vi "removeStiff.vi"() -> ()   [LabVIEW 2015]
uses:
  GlobalPath.vi
  GlobalData.vi
  GlobalVi.vi
panel:
  in  "ptfe 6":bool caption="Move the stiffback away from the panel"
  in  "ptfe 5":bool caption="Lift the stiffback from the panel"
  in  "Done ?":bool
  in  "ptfe 4":bool caption="Connect the stiffback to the movement arch"
  in  "ptfe 3":bool caption="Remove the weights placed on the panel"
  in  "ptfe 2":bool caption="Stop the table vacuum"
  # "Stiffback Removal"
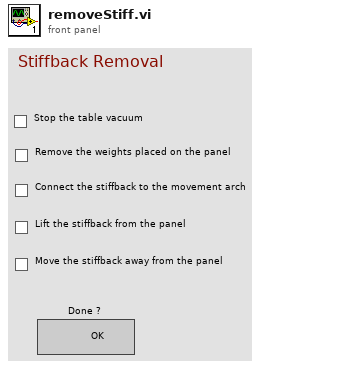
[diagram p1: front panel]
types:
  T1 = enum16{"open", "replace", "create", "open or create", "replace or create", "replace or create with confirmation"}
  T2 = enum32{"Bad", "Idle", "Run top level", "Running"}
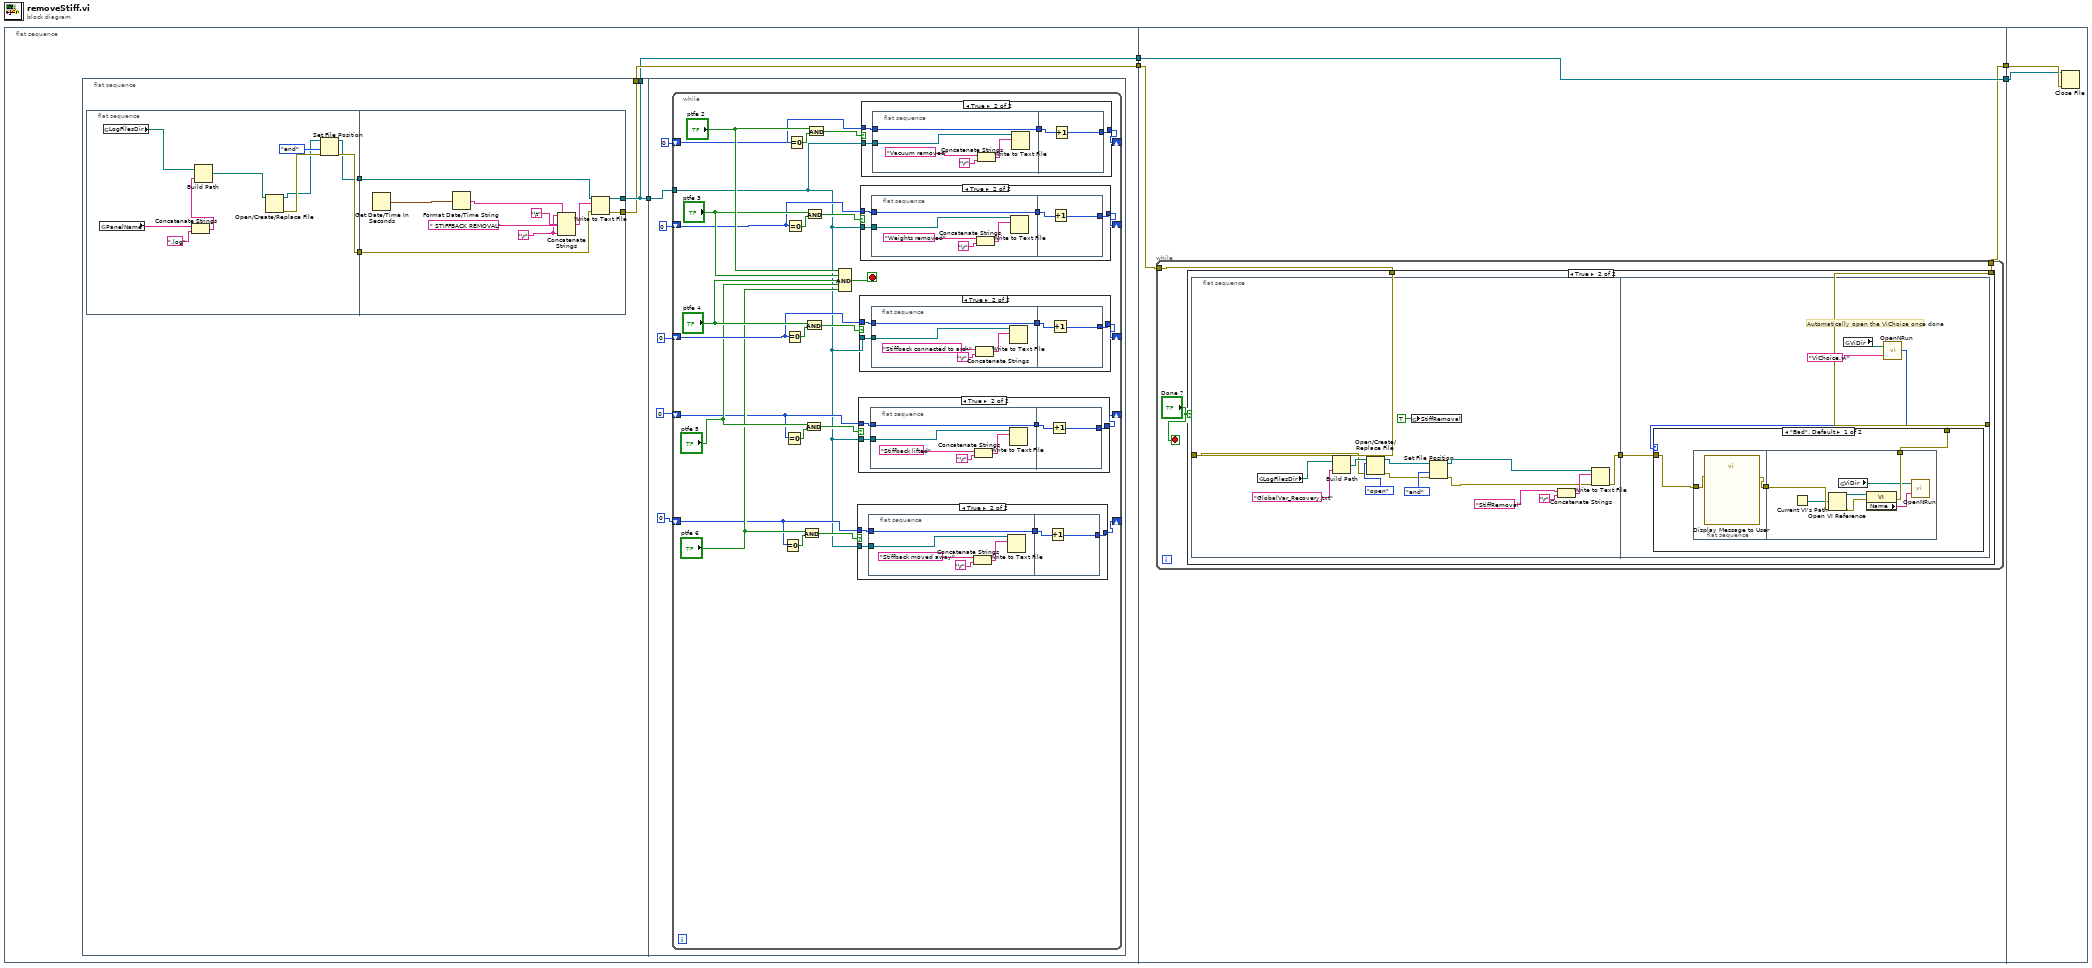
[diagram p0: block diagram]
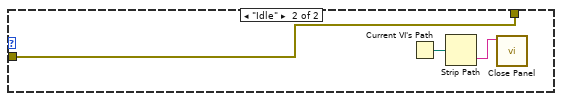
[diagram p8: hidden frame]
diagram:
  n1 = flat-sequence {
    tunnel: [w6] -> w3
    tunnel: [w5] -> w2
    tunnel: [w126] -> w4
    tunnel: w3 -> [w125]
    tunnel: w2 -> [w127]
    tunnel: [w127] -> w1
    tunnel: w4 -> [w171]
    tunnel: w1 -> [w170]
    frame #0 {
      n2 = flat-sequence {
        tunnel: [w10] -> w7
        tunnel: [w10] -> w5
        tunnel: [w9] -> w6
        tunnel: w7 -> [w37]
        frame #0 {
          n3 = flat-sequence {
            tunnel: [w13] -> w11
            tunnel: [w15] -> w8
            tunnel: w11 -> [w27]
            tunnel: [w26] -> w10
            tunnel: [w25] -> w9
            tunnel: w8 -> [w24]
            frame #0 {
              n4 = global read "GlobalData.vi" "PanelName"() -> (w20:string)
              n5 = global read "GlobalPath.vi" "LogFilesDir"() -> (w12:path)
              n6 = Concatenate Strings(w20, ".log") -> (w19:string)
              n7 = Build Path(base path=w12, name or relative path=w19) -> (appended path=w18:path)
              n8 = Open/Create/Replace File(file path (use dialog)=w18) -> (refnum out=w14:refnum<file>, error out=w16:errorcluster)  [unwired: 5 in, 1 out]
              n9 = Set File Position(refnum=w14, from (0:start)=enum16{"start", "end", "current"}."end", error in=w16) -> (refnum out=w13:refnum<file>, error out=w15:errorcluster)  [unwired: 1 in]
            }
            frame #1 {
              w22 = "\r"
              n10 = Get Date/Time In Seconds() -> (seconds since 1Jan1904=w23:timestamp)
              n11 = Format Date/Time String(seconds (now)=w23) -> (date/time string=w29:string)  [unwired: 2 in]
              n12 = Concatenate Strings(w22, w29, "\t", " STIFFBACK REMOVAL", w22) -> (w28:string)
              n13 = Write to Text File(file (use dialog)=w27, text=w28, error in=w24) -> (refnum out=w26:refnum<file>, error out=w25:errorcluster)  [unwired: 1 in, 1 out]
            }
          }
        }
        frame #1 {
          n14 = while {
            tunnel: w37 -> [w38]
            shift-right: [w55] -> _
            shift-left: 0 -> [w60]
            shift-right: [w54] -> _
            shift-left: 0 -> [w56]
            shift-right: [w49] -> _
            shift-left: 0 -> [w50]
            shift-right: [w40] -> _
            shift-left: 0 -> [w42]
            shift-right: [w39] -> _
            shift-left: 0 -> [w41]
            stop <- w64 stop-if-true
            n15 = Equal To 0?(x=w42) -> (x = 0?=w46:bool)
            n16 = Equal To 0?(x=w41) -> (x = 0?=w48:bool)
            n17 = Equal To 0?(x=w50) -> (x = 0?=w53:bool)
            n18 = Equal To 0?(x=w56) -> (x = 0?=w59:bool)
            n19 = Equal To 0?(x=w60) -> (x = 0?=w63:bool)
            n20 = And(x="ptfe 6", y=w46) -> (x .and. y?=w45:bool)
            n21 = And(x="ptfe 5", y=w48) -> (x .and. y?=w47:bool)
            n22 = And(x="ptfe 4", y=w53) -> (x .and. y?=w52:bool)
            n23 = And(x="ptfe 3", y=w59) -> (x .and. y?=w58:bool)
            n24 = And(x="ptfe 2", y=w63) -> (x .and. y?=w62:bool)
            n25 = Compound Arithmetic op=AND("ptfe 2", "ptfe 3", "ptfe 4", "ptfe 5", "ptfe 6") -> (w64:bool)
            n26 = case shown="True" w45 {
              tunnel: w38 -> [_ w69]
              tunnel: w42 -> [w65 w67]
              tunnel: [w65 w66] -> w40
              frame False {
              }
              frame True {
                n27 = flat-sequence {
                  tunnel: w69 -> [w72]
                  tunnel: [w71] -> w68
                  tunnel: w67 -> [w71]
                  tunnel: w68 -> [w76]
                  tunnel: [w75] -> w66
                  frame #0 {
                    n28 = Concatenate Strings("Stiffback moved away", "\r") -> (w74:string)
                    n29 = Write to Text File(file (use dialog)=w72, text=w74) -> ()  [unwired: 2 in, 3 out]
                  }
                  frame #1 {
                    n30 = Increment(x=w76) -> (x+1=w75:i32)
                  }
                }
              }
            }
            n31 = case shown="True" w47 {
              tunnel: w38 -> [_ w81]
              tunnel: w41 -> [w77 w79]
              tunnel: [w77 w78] -> w39
              frame False {
              }
              frame True {
                n32 = flat-sequence {
                  tunnel: w81 -> [w84]
                  tunnel: [w83] -> w80
                  tunnel: w79 -> [w83]
                  tunnel: w80 -> [w88]
                  tunnel: [w87] -> w78
                  frame #0 {
                    n33 = Concatenate Strings("Stiffback lifted", "\r") -> (w86:string)
                    n34 = Write to Text File(file (use dialog)=w84, text=w86) -> ()  [unwired: 2 in, 3 out]
                  }
                  frame #1 {
                    n35 = Increment(x=w88) -> (x+1=w87:i32)
                  }
                }
              }
            }
            n36 = case shown="True" w52 {
              tunnel: w38 -> [_ w93]
              tunnel: w50 -> [w89 w91]
              tunnel: [w89 w90] -> w49
              frame False {
              }
              frame True {
                n37 = flat-sequence {
                  tunnel: w93 -> [w96]
                  tunnel: [w95] -> w92
                  tunnel: w91 -> [w95]
                  tunnel: w92 -> [w100]
                  tunnel: [w99] -> w90
                  frame #0 {
                    n38 = Concatenate Strings("Stiffback connected to arch", "\r") -> (w98:string)
                    n39 = Write to Text File(file (use dialog)=w96, text=w98) -> ()  [unwired: 2 in, 3 out]
                  }
                  frame #1 {
                    n40 = Increment(x=w100) -> (x+1=w99:i32)
                  }
                }
              }
            }
            n41 = case shown="True" w58 {
              tunnel: w38 -> [_ w105]
              tunnel: w56 -> [w101 w103]
              tunnel: [w101 w102] -> w54
              frame False {
              }
              frame True {
                n42 = flat-sequence {
                  tunnel: w105 -> [w108]
                  tunnel: [w107] -> w104
                  tunnel: w103 -> [w107]
                  tunnel: w104 -> [w112]
                  tunnel: [w111] -> w102
                  frame #0 {
                    n43 = Concatenate Strings("Weights removed", "\r") -> (w110:string)
                    n44 = Write to Text File(file (use dialog)=w108, text=w110) -> ()  [unwired: 2 in, 3 out]
                  }
                  frame #1 {
                    n45 = Increment(x=w112) -> (x+1=w111:i32)
                  }
                }
              }
            }
            n46 = case shown="True" w62 {
              tunnel: w38 -> [_ w117]
              tunnel: w60 -> [w113 w115]
              tunnel: [w113 w114] -> w55
              frame False {
              }
              frame True {
                n47 = flat-sequence {
                  tunnel: w117 -> [w120]
                  tunnel: [w119] -> w116
                  tunnel: w115 -> [w119]
                  tunnel: w116 -> [w124]
                  tunnel: [w123] -> w114
                  frame #0 {
                    n48 = Concatenate Strings("Vacuum removed", "\r") -> (w122:string)
                    n49 = Write to Text File(file (use dialog)=w120, text=w122) -> ()  [unwired: 2 in, 3 out]
                  }
                  frame #1 {
                    n50 = Increment(x=w124) -> (x+1=w123:i32)
                  }
                }
              }
            }
          }
        }
      }
    }
    frame #1 {
      n51 = while {
        tunnel: [w129] -> w126
        tunnel: w125 -> [w128]
        stop <- "Done ?" stop-if-true
        n52 = case shown="True" "Done ?" {
          tunnel: [w131 w133] -> w129
          tunnel: w128 -> [w131 w132]
          frame False {
          }
          frame True {
            n53 = flat-sequence {
              tunnel: w132 -> [w138]
              tunnel: [w137] -> w134
              tunnel: [w151] -> w133
              tunnel: w134 -> [w150]
              frame #0 {
                n54 = global read "GlobalPath.vi" "LogFilesDir"() -> (w135:path)
                n55 = Build Path(base path=w135, name or relative path="GlobalVar_Recovery.txt") -> (appended path=w147:path)
                n56 = Open/Create/Replace File(file path (use dialog)=w147, error in=w138, operation (0:open)=T1."open") -> (refnum out=w143:refnum<file>, error out=w144:errorcluster)  [unwired: 3 in, 1 out]
                n57 = global write "GlobalVi.vi" "StiffRemoval"(TRUE) -> ()
                n58 = Set File Position(refnum=w143, from (0:start)=enum16{"start", "end", "current"}."end", error in=w144) -> (refnum out=w140:refnum<file>, error out=w139:errorcluster)  [unwired: 1 in]
                n59 = Concatenate Strings("StiffRemoval", "\r") -> (w142:string)
                n60 = Write to Text File(file (use dialog)=w140, text=w142, error in=w139) -> (error out=w137:errorcluster)  [unwired: 1 in, 2 out]
              }
              frame #1 {
                # "Automatically open the ViChoise once done"
                n61 = global read "GlobalPath.vi" "ViDir"() -> (w154:path)
                n62 = call "OpenNRun.vi"("VI name"="ViChoice.vi", "ViDirPath"=w154) -> ("Execution:State"=w153:T2)
                n63 = case shown="\"Bad\", Default" w153 {
                  tunnel: [w155 w167] -> w151
                  tunnel: w150 -> [w156 w167]
                  frame "Bad", Default {
                    n64 = flat-sequence {
                      tunnel: w156 -> [w159]
                      tunnel: [w158] -> w157
                      tunnel: [w163] -> w155
                      tunnel: w157 -> [w162]
                      frame #0 {
                        n65 = call "Display Message to User"("error in (no error)"=w159) -> ("error out"=w158:errorcluster)  [unwired: 9 in, 1 out]
                      }
                      frame #1 {
                        n66 = Current VI's Path() -> (path=w160:path)
                        n67 = Open VI Reference(vi path=w160, error in (no error)=w162) -> (vi reference=w166:refnum<vi>, error out=w165:errorcluster)  [unwired: 4 in]
                        n68 = global read "GlobalPath.vi" "ViDir"() -> (w161:path)
                        n69 = property class="VI"(reference=w166, error in=w165) -> (error out=w163:errorcluster, "Name"=w164:string)  [unwired: 1 out]
                        n70 = call "OpenNRun.vi"("VI name"=w164, "ViDirPath"=w161) -> ()  [unwired: 1 out]
                      }
                    }
                  }
                  frame "Idle" {
                    n71 = Current VI's Path() -> (path=w168:path)
                    n72 = Strip Path(path=w168) -> (name=w169:string)  [unwired: 1 out]
                    n73 = call <vilib>:"Close Panel.vi"("VI name"=w169) -> ()  [unwired: 10 in, 1 out]
                  }
                }
              }
            }
          }
        }
      }
    }
    frame #2 {
      n74 = Close File(refnum=w170, error in=w171) -> ()  [unwired: 2 out]
    }
  }
